vi "CH_LM Action Probe Zero.vi"(0 "Meter Index":i32, 5 "error in (no error)":errorcluster, 7 "Timeout / ms (3000)":i32=3000, 8 "Action (query)":bool, 9 "Lock Timeout / ms (1000)":i32=1000) -> (11 "Lock timed out":bool, 14 "Meter Index":i32, 15 "Zero Offset / W":dbl format="%#.3g", 19 "error out":errorcluster)   [LabVIEW 2012, in "CH_LM.lvlib"]
doc: "This command will set the current probe input voltage as the zero baseline voltage. If a valid thermopile or optical probe is attached, the probe will be zeroed for all usable ranges if auto ranging is active and will be zeroed for the current range if auto ranging is not active. This command will have result in no internal action taken if a pyroelectric probe is attached or if a valid probe is not attached.\n\nThe zero query will return the offset in Watts used to generate the zeroed output if a valid thermopile or optical probe is attached. Otherwise, 0 will be returned."
uses:
  CH_LM.lvlib
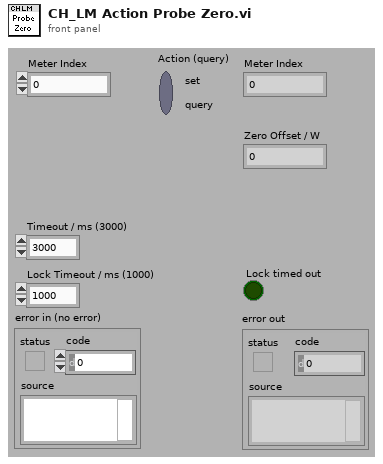
[diagram p1: front panel]
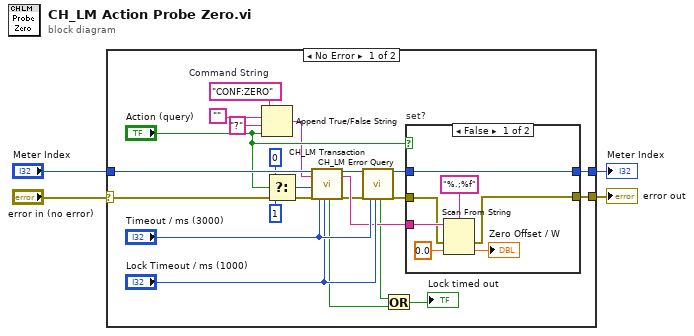
[diagram p0: block diagram]
diagram:
  n1 = case shown="No Error" "error in (no error)" {
    selector: "error in (no error)" -> [w26 w37]
    tunnel: [w24 w37] -> w4
    tunnel: "Meter Index" -> [w25 w36]
    tunnel: [w23 w36] -> w1
    frame No Error {
      w19 = "CONF:ZERO"  # Command String
      n2 = Append True/False String(1:"Action (query)", 2:"?" ("true string"), 3:"", 4:w19) -> (0:w6:string)
      n3 = Select(t=0, s="Action (query)", f=1 ("NofStrings (-1:all)")) -> (s? t:f=w15:i32)
      n4 = call "CH_LM Transaction.vi"("Meter Index"=w25, "Command String"=w6, "NofStrings (-1:all)"=w15, "error in (no error)"=w26, "Timeout / ms (3000)"="Timeout / ms (3000)", "Lock Timeout / ms (1000)"="Lock Timeout / ms (1000)") -> ("Lock timed out"=w8:bool, "Meter Index"=w13:i32, "Response"=w18:string, "error out"=w11:errorcluster)  [unwired: 10 out]
      n5 = call "CH_LM Error Query.vi"("Meter Index"=w13, "error in (no error)"=w11, "Timeout / ms (3000)"="Timeout / ms (3000)", "Lock Timeout / ms (1000)"="Lock Timeout / ms (1000)") -> ("Lock timed out"=w9:bool, "Meter Index"=w12:i32, "error out"=w10:errorcluster)  [unwired: 13 out]
      n6 = Or(x=w9, y=w8) -> (x .or. y?=→"Lock timed out":bool)
      n7 = case "set?" shown="False" "Action (query)" {
        tunnel: w18 -> [w33 _]
        tunnel: w10 -> [w32 w35]
        tunnel: [w31 w35] -> w24
        tunnel: w12 -> [w27 w34]
        tunnel: [w27 w34] -> w23
        frame False {
          n8 = Scan From String(format string="%.;%f", input string=w33, error in=w32, default 1=0.0 ("default value 1")) -> (error out=w31:errorcluster, output 1=→"Zero Offset / W":dbl)  [unwired: 1 in, 2 out]
        }
        frame True {
        }
      }
    }
    frame Error {
    }
  }
  "error out" <- w4
  "Meter Index" <- w1
